vi "SubVI_getSpectra.vi"(1 "endPix":u16=3652, 2 "startPix":u16, 3 "test1":u8, 5 "Fast":u8, 7 "trigger":bool, 8 "keep trigger":bool, 9 "blank scans number":u8, 10 "scans number":u8=1, 11 "Exposure":u16=2) -> (0 "all spectra":i16[][](array[numeric]), 4 "Error":bool)   [LabVIEW 2022 SP3]
uses:
  adcDLL_0001.dll
panel:
  out "test count":i32
  in  "tot_startPix":u16=33
  in  "tot_endPix":u16=3685
  out "CountExposure":u16
  out "Count blanc":u8
  out "CountScans":u8
  out "program\nin process":bool
  out "Spectra 2":i16[](array[numeric])
  out "Spectra":i16[](array[numeric])
  out "InputReport1":u8[](array[numeric]) format="%x"
  out "Output Report":u8[](array[numeric])
  out "Input Report":u8[](array[numeric])
  # "test1 - \"1\" returne 0- 3711 (116*32)\n            \"0\" returne according to below\nFast -   \"0\" every pixel\n            \"1\" one out of 2 pixels in useful\n            information range"
  # "Move SRAM\ncount"
  # "384"
  # "useful information is in this range \n(already inside range of useful information)"
  # "useful information is in this range"
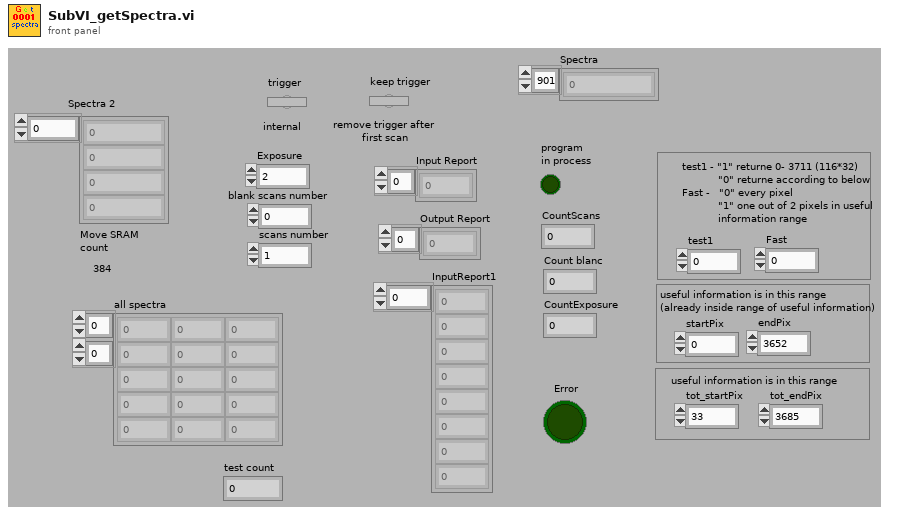
[diagram p1: front panel]
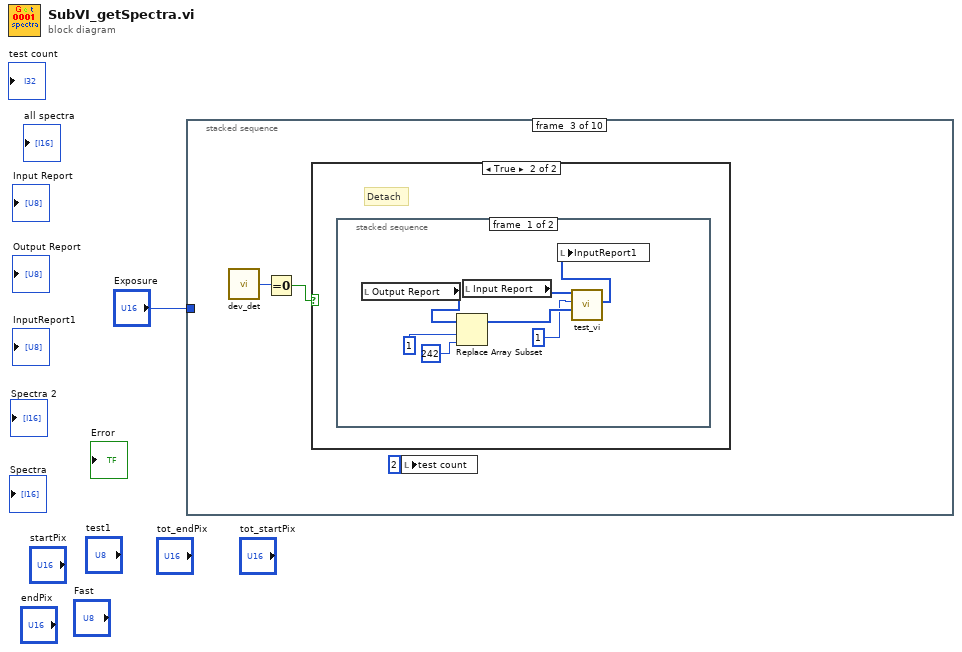
[diagram p0: block diagram]
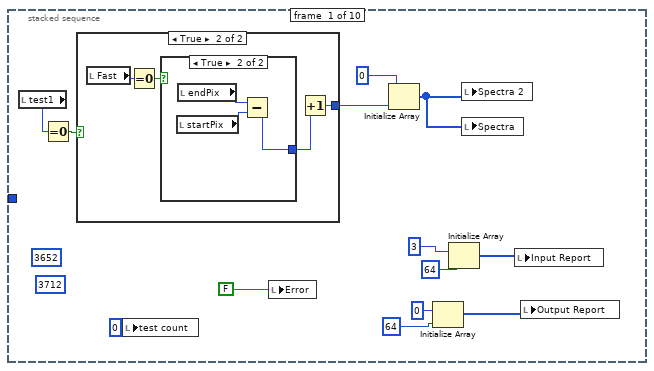
[diagram p2: hidden frame]
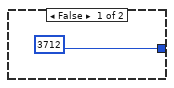
[diagram p3: hidden frame]
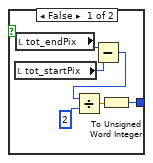
[diagram p4: hidden frame]
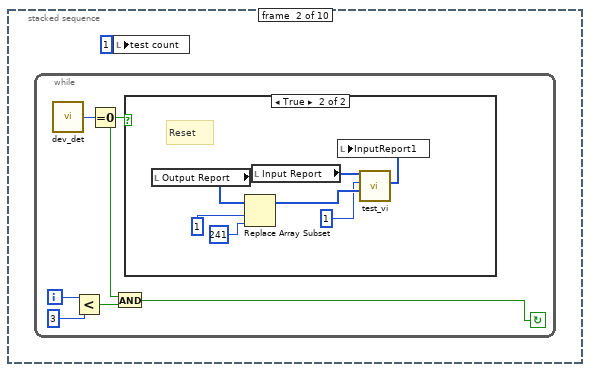
[diagram p5: hidden frame]
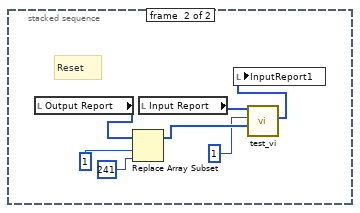
[diagram p8: hidden frame]
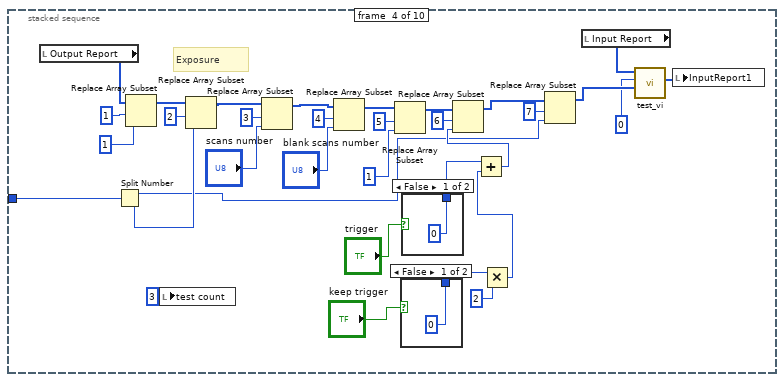
[diagram p9: hidden frame]
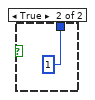
[diagram p10: hidden frame]
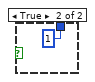
[diagram p11: hidden frame]
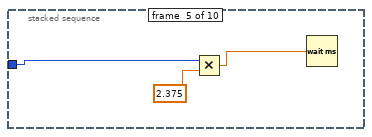
[diagram p12: hidden frame]
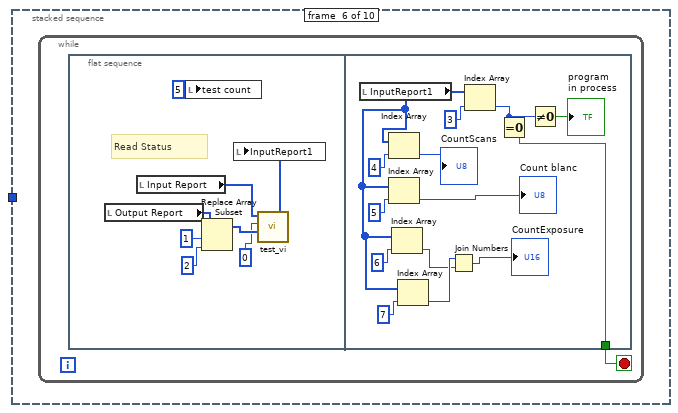
[diagram p13: hidden frame]
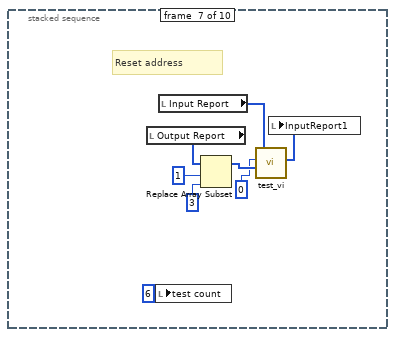
[diagram p14: hidden frame]
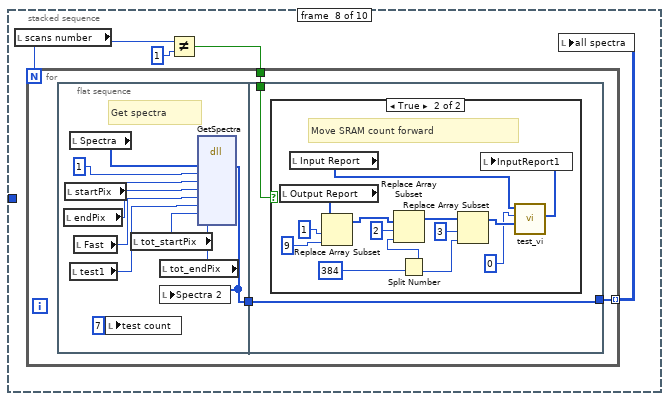
[diagram p15: hidden frame]
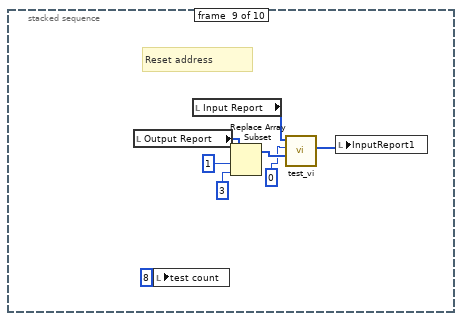
[diagram p17: hidden frame]
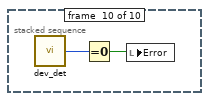
[diagram p18: hidden frame]
diagram:
  n1 = stacked-sequence {
    tunnel: "Exposure" -> [_ _ _ w63 w99 _ _ _ _ _]
    frame #0 {
      (unwired) u16 3712
      (unwired) 3652 ("dimension size")
      n2 = local read "test1"() -> (w6:u8)
      n3 = Equal To 0?(x=w6) -> (x = 0?=w5:bool)
      n4 = case shown="True" w5 {
        tunnel: [u16 3712 w16] -> w4
        frame False {
        }
        frame True {
          n5 = local read "Fast"() -> (w19:u8)
          n6 = Equal To 0?(x=w19) -> (x = 0?=w18:bool)
          n7 = case shown="True" w18 {
            tunnel: [w23 w28] -> w17
            frame False {
              n8 = local read "tot_startPix"() -> (w22:u16)
              n9 = local read "tot_endPix"() -> (w21:u16)
              n10 = Subtract(x=w21, y=w22) -> (x-y=w20:u16)
              n11 = Divide(x=w20, y=u16 2) -> (x/y=w24:dbl)
              n12 = To Unsigned Word Integer(number=w24) -> (unsigned 16bit integer=w23:u16)
            }
            frame True {
              n13 = local read "startPix"() -> (w26:u16)
              n14 = local read "endPix"() -> (w27:u16)
              n15 = Subtract(x=w27, y=w26) -> (x-y=w28:u16)
            }
          }
          n16 = Increment(x=w17) -> (x+1=w16:u16)
        }
      }
      n17 = local write "test count"(0 ("test count")) -> ()
      n18 = local write "Error"(FALSE ("Boolean")) -> ()
      n19 = Initialize Array(u16 0 ("element"), w4) -> (w13:u16[])
      n20 = Initialize Array(u8 0 ("element"), 64 ("dimension size")) -> (w7:u8[])
      n21 = Initialize Array(u8 3 ("element"), 64 ("dimension size")) -> (w8:u8[])
      n22 = local write "Spectra 2"(w13) -> ()
      n23 = local write "Spectra"(w13) -> ()
      n24 = local write "Input Report"(w8) -> ()
      n25 = local write "Output Report"(w7) -> ()
    }
    frame #1 {
      n26 = while {
        i -> [w34]
        stop <- w30 continue-if-true
        n27 = call "dev_det.vi"() -> ("DevDetect 2"=w35:u8)
        n28 = Less?(x=w34, y=3) -> (x < y?=w32:bool)
        n29 = Equal To 0?(x=w35) -> (x = 0?=w31:bool)
        n30 = And(x=w31, y=w32) -> (x .and. y?=w30:bool)
        n31 = case shown="True" w31 {
          frame False {
          }
          frame True {
            # "Reset"
            n32 = local read "Output Report"() -> (w40:u8[])
            n33 = Replace Array Subset(array=w40, new element=u8 241 ("new element/subarray"), index=1) -> (w41:u8[])
            n34 = local read "Input Report"() -> (w39:u8[])
            n35 = call "test_vi.vi"("OutputReport_in"=w41, "DevDet_in"=1, "InputReport_in"=w39) -> ("InputReport_out"=w42:u8[])  [unwired: 1 in, 3 out]
            n36 = local write "InputReport1"(w42) -> ()
          }
        }
      }
      n37 = local write "test count"(1 ("test count")) -> ()
    }
    frame #2 {
      n38 = call "dev_det.vi"() -> ("DevDetect 2"=w45:u8)
      n39 = Equal To 0?(x=w45) -> (x = 0?=w44:bool)
      n40 = case shown="True" w44 {
        frame False {
        }
        frame True {
          # "Detach"
          n41 = stacked-sequence {
            frame #0 {
              n42 = local read "Output Report"() -> (w50:u8[])
              n43 = Replace Array Subset(array=w50, new element=u8 242 ("new element/subarray"), index=1) -> (w47:u8[])
              n44 = local read "Input Report"() -> (w51:u8[])
              n45 = call "test_vi.vi"("OutputReport_in"=w47, "DevDet_in"=1, "InputReport_in"=w51) -> ("InputReport_out"=w52:u8[])  [unwired: 1 in, 3 out]
              n46 = local write "InputReport1"(w52) -> ()
            }
            frame #1 {
              # "Reset"
              n47 = local read "Output Report"() -> (w57:u8[])
              n48 = Replace Array Subset(array=w57, new element=u8 241 ("new element/subarray"), index=1) -> (w54:u8[])
              n49 = local read "Input Report"() -> (w58:u8[])
              n50 = call "test_vi.vi"("OutputReport_in"=w54, "DevDet_in"=1, "InputReport_in"=w58) -> ("InputReport_out"=w59:u8[])  [unwired: 1 in, 3 out]
              n51 = local write "InputReport1"(w59) -> ()
            }
          }
        }
      }
      n52 = local write "test count"(2 ("test count")) -> ()
    }
    frame #3 {
      # "Exposure"
      n53 = local read "Output Report"() -> (w90:u8[])
      n54 = Split Number(x=w63) -> (hi(x)=w62:u8, lo(x)=w64:u8)
      n55 = Replace Array Subset(array=w90, new element=u8 1 ("new element/subarray"), index=1) -> (w92:u8[])
      n56 = local write "test count"(3 ("test count")) -> ()
      n57 = Replace Array Subset(array=w92, new element=w64, index=2) -> (w84:u8[])
      n58 = Replace Array Subset(array=w84, new element="scans number", index=3) -> (w81:u8[])
      n59 = Replace Array Subset(array=w81, new element="blank scans number", index=4) -> (w79:u8[])
      n60 = Replace Array Subset(array=w79, new element=1 ("index"), index=5) -> (w75:u8[])
      n61 = case shown="False" "keep trigger" {
        tunnel: [0 ("index") 1 ("index")] -> w71
        frame False {
        }
        frame True {
        }
      }
      n62 = case shown="False" "trigger" {
        tunnel: [0 ("index") 1 ("index")] -> w69
        frame False {
        }
        frame True {
        }
      }
      n63 = Multiply(x=w71, y=2 ("index")) -> (x*y=w70:i32)
      n64 = Add(x=w69, y=w70) -> (x+y=w68:i32)
      n65 = Replace Array Subset(array=w75, new element=w68, index=6) -> (w65:u8[])
      n66 = Replace Array Subset(array=w65, new element=w62, index=7) -> (w61:u8[])
      n67 = local read "Input Report"() -> (w87:u8[])
      n68 = call "test_vi.vi"("OutputReport_in"=w61, "DevDet_in"=0, "InputReport_in"=w87) -> ("InputReport_out"=w86:u8[])  [unwired: 1 in, 3 out]
      n69 = local write "InputReport1"(w86) -> ()
    }
    frame #4 {
      n70 = Multiply(x=w99, y=2.375) -> (x*y=w97:dbl)
      n71 = Wait (ms)(milliseconds to wait=w97) -> ()  [unwired: 1 out]
    }
    frame #5 {
      n72 = while {
        stop <- w100 stop-if-true
        n73 = flat-sequence {
          tunnel: [w121] -> w100
          frame #0 {
            # "Read Status"
            n74 = local read "Output Report"() -> (w106:u8[])
            n75 = local read "Input Report"() -> (w107:u8[])
            n76 = local write "test count"(5 ("test count")) -> ()
            n77 = Replace Array Subset(array=w106, new element=u8 2 ("new element/subarray"), index=1) -> (w102:u8[])
            n78 = call "test_vi.vi"("OutputReport_in"=w102, "DevDet_in"=0, "InputReport_in"=w107) -> ("InputReport_out"=w108:u8[])  [unwired: 1 in, 3 out]
            n79 = local write "InputReport1"(w108) -> ()
          }
          frame #1 {
            n80 = local read "InputReport1"() -> (w112:u8[])
            n81 = Index Array(array=w112, index=4) -> (element=→"CountScans":u8)
            n82 = Index Array(array=w112, index=5) -> (element=→"Count blanc":u8)
            n83 = Index Array(array=w112, index=6) -> (element=w110:u8)
            n84 = Index Array(array=w112, index=7) -> (element=w111:u8)
            n85 = Join Numbers(hi=w111, lo=w110) -> ((hi.lo)=→"CountExposure":u16)
            n86 = Index Array(array=w112, index=3) -> (element=w120:u8)
            n87 = Equal To 0?(x=w120) -> (x = 0?=w121:bool)
            n88 = Not Equal To 0?(x=w120) -> (x != 0?=→"program\nin process":bool)
          }
        }
      }
    }
    frame #6 {
      # "Reset address"
      n89 = local read "Output Report"() -> (w128:u8[])
      n90 = local write "test count"(6 ("test count")) -> ()
      n91 = local read "Input Report"() -> (w129:u8[])
      n92 = Replace Array Subset(array=w128, new element=u8 3 ("new element/subarray"), index=1) -> (w124:u8[])
      n93 = call "test_vi.vi"("OutputReport_in"=w124, "DevDet_in"=0, "InputReport_in"=w129) -> ("InputReport_out"=w130:u8[])  [unwired: 1 in, 3 out]
      n94 = local write "InputReport1"(w130) -> ()
    }
    frame #7 {
      n95 = local read "scans number"() -> (w132:u8)
      n96 = Not Equal?(x=w132, y=u8 1) -> (x != y?=w131:bool)
      n97 = for {
        N: w132 -> [_]
        tunnel: [w137] -> w134 mode=indexing
        tunnel: w131 -> [w135]
        n98 = flat-sequence {
          tunnel: [w147] -> w136
          tunnel: [w149] -> w137
          tunnel: w136 -> [w149]
          tunnel: w135 -> [w148]
          frame #0 {
            # "Get spectra"
            n99 = local read "endPix"() -> (w143:u16)
            n100 = local read "startPix"() -> (w144:u16)
            n101 = local read "Spectra"() -> (w146:i16[])
            n102 = local read "test1"() -> (w141:u8)
            n103 = local read "Fast"() -> (w142:u8)
            n104 = local write "test count"(7 ("test count")) -> ()
            n105 = local read "tot_startPix"() -> (w139:u16)
            n106 = local read "tot_endPix"() -> (w140:u16)
            n107 = dll-call lib="D:/LabVIEWSuite_64_OS/Spectrometers/ASEQ LR1/adcDLL_0001.dll" fn="GetSpectra"("InputSpec1"=w146, "SpecNmb"=u8 1, "startPix"=w144, "endPix"=w143, "Fast"=w142, "test1"=w141, "tot_startPix"=w139, "tot_endPix"=w140) -> ("InputSpec1"=w147:i16[])  [unwired: 11 in, 2 out]
            n108 = local write "Spectra 2"(w147) -> ()
          }
          frame #1 {
            n109 = case shown="True" w148 {
              frame False {
              }
              frame True {
                # "Move SRAM count forward"
                n110 = local read "Output Report"() -> (w163:u8[])
                n111 = local read "Input Report"() -> (w160:u8[])
                n112 = Replace Array Subset(array=w163, new element=u8 9 ("new element/subarray"), index=1) -> (w156:u8[])
                n113 = Split Number(x=u16 384) -> (hi(x)=w157:u8, lo(x)=w154:u8)
                n114 = Replace Array Subset(array=w156, new element=w157, index=2) -> (w153:u8[])
                n115 = Replace Array Subset(array=w153, new element=w154, index=3) -> (w151:u8[])
                n116 = call "test_vi.vi"("OutputReport_in"=w151, "DevDet_in"=0, "InputReport_in"=w160) -> ("InputReport_out"=w159:u8[])  [unwired: 1 in, 3 out]
                n117 = local write "InputReport1"(w159) -> ()
              }
            }
          }
        }
      }
      n118 = local write "all spectra"(w134) -> ()
    }
    frame #8 {
      # "Reset address"
      n119 = local read "Output Report"() -> (w170:u8[])
      n120 = local write "test count"(8 ("test count")) -> ()
      n121 = local read "Input Report"() -> (w169:u8[])
      n122 = Replace Array Subset(array=w170, new element=u8 3 ("new element/subarray"), index=1) -> (w165:u8[])
      n123 = call "test_vi.vi"("OutputReport_in"=w165, "DevDet_in"=0, "InputReport_in"=w169) -> ("InputReport_out"=w171:u8[])  [unwired: 1 in, 3 out]
      n124 = local write "InputReport1"(w171) -> ()
    }
    frame #9 {
      n125 = call "dev_det.vi"() -> ("DevDetect 2"=w173:u8)
      n126 = Equal To 0?(x=w173) -> (x = 0?=w172:bool)
      n127 = local write "Error"(w172) -> ()
    }
  }
